vi "FitsCreateImage.vi"(6 "naxes":i64[](array[numeric]), 8 "error in (no error)":errorcluster, 9 "naxis":i32, 10 "ref in":u64, 11 "CFitsIO in":refnum<class "CFitsIO.lvclass">) -> (0 "error out":errorcluster, 2 "ref out":u64, 3 "CFitsIO out":refnum<class "CFitsIO.lvclass">)   [LabVIEW 2016, in "CFitsIO.lvclass"]
uses:
  CFitsIO.lvclass
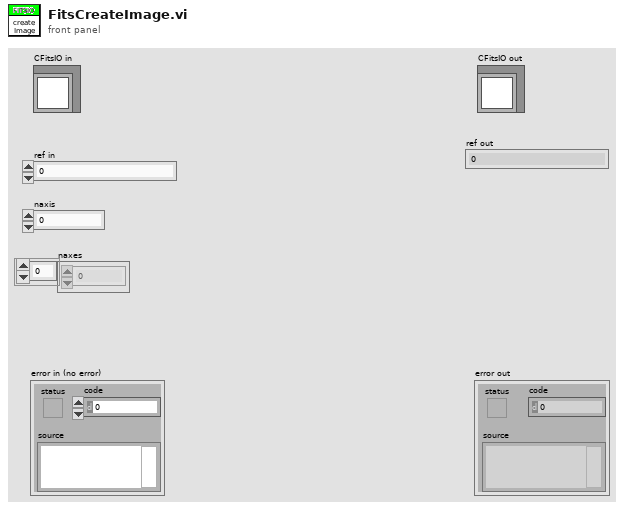
[diagram p1: front panel]
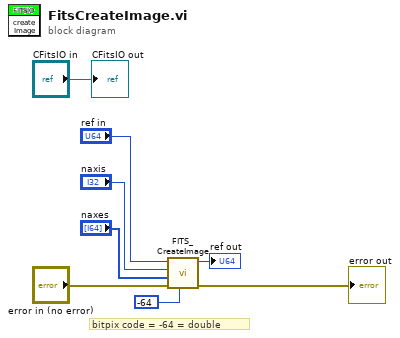
[diagram p0: block diagram]
diagram:
  # "bitpix code = -64 = double"
  n1 = call "FITS_CreateImage.vi"("bitpix code"=-64, "error in"="error in (no error)", "naxes"="naxes", "naxis"="naxis", "ref in"="ref in") -> ("error out"=→"error out":errorcluster, "ref out"=→"ref out":u64)  [unwired: 5 in]
  "CFitsIO out" <- "CFitsIO in"
